vi "set results reporter.vi"(10 "results reporter":refnum<class "results reporter.lvclass">, 11 "task in":refnum<class "task.lvclass">) -> (3 "task out":refnum<class "task.lvclass">)   [LabVIEW 2013, in "task.lvclass"]
uses:
  task.lvclass
  results reporter/results reporter.lvclass
  task.lvclass/task.ctl
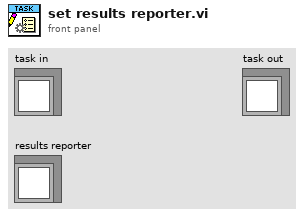
[diagram p1: front panel]
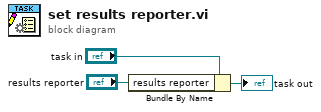
[diagram p0: block diagram]
diagram:
  n1 = Bundle By Name(cluster="task in", "results reporter"="results reporter") -> (→"task out":refnum<class "task.lvclass">)
